vi "putAPointAsObstacleInPotentialField.vi"(6 "ArrayOfObstacles in":T1[](array[typedef]), 9 "multiplier":dbl, 10 "influence radius":dbl, 11 "point":dbl[](array[numeric])) -> (3 "ArrayOfObstacles out":T1[](array[typedef]))   [LabVIEW 2023, in "Robot.lvclass"]
uses:
  Robot.lvclass
  obstacle.ctl
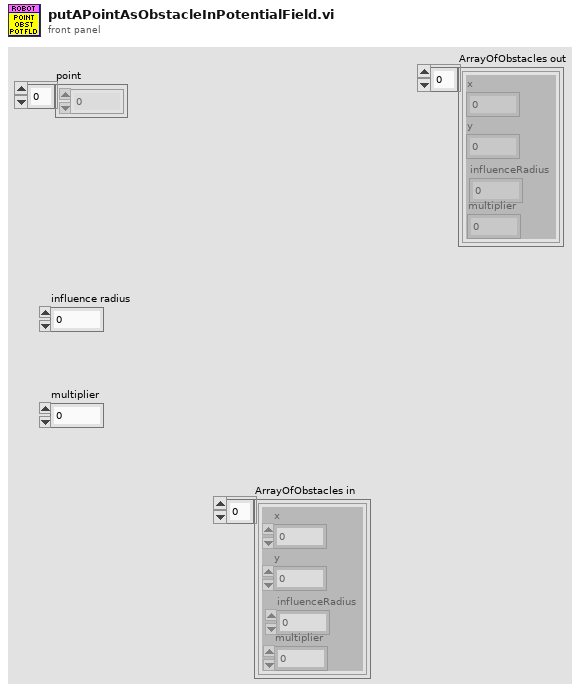
[diagram p1: front panel]
types:
  T1 = typedef "obstacle.ctl" = cluster{"x":dbl, "y":dbl, "influenceRadius":dbl, "multiplier":dbl}
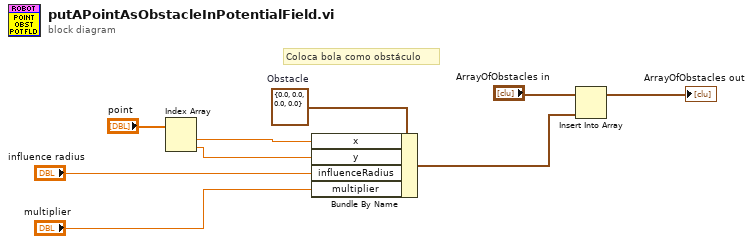
[diagram p0: block diagram]
diagram:
  w4 = T1 {"x"=0.0, "y"=0.0, "influenceRadius"=0.0, "multiplier"=0.0}  # Obstacle
  # "Coloca bola como obstáculo"
  n1 = Index Array(array="point") -> (element #1=w2:dbl, element #2=w1:dbl)  [unwired: 2 in]
  n2 = Bundle By Name(cluster=w4, "x"=w2, "y"=w1, "influenceRadius"="influence radius", "multiplier"="multiplier") -> (w6:T1)
  n3 = Insert Into Array(array="ArrayOfObstacles in", new element=w6) -> (→"ArrayOfObstacles out":T1[])  [unwired: 1 in]
